vi "Main.vi"(8 "error in (no error)":errorcluster, 9 "Port":u16=4663, 10 "Run External":bool, 11 "Control VI":T1) -> (0 "error out":errorcluster)   [LabVIEW 2024, in "FormulaG.lvlib" / "FormulaG App.lvclass"]
uses:
  FormulaG App.lvclass
  FormulaG-Common/Control VI.ctl
  FormulaG-Common/FormulaG-Common.lvlib
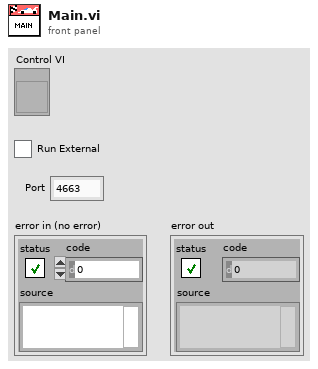
[diagram p1: front panel]
types:
  T1 = typedef "FormulaG-Common.lvlib/Control VI.ctl" = refnum<vi>
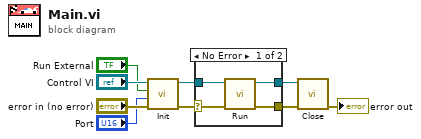
[diagram p0: block diagram]
diagram:
  n1 = call "Init.vi"("error in (no error)"="error in (no error)", "Port"="Port", "Run External"="Run External", "Control VI"="Control VI") -> ("error out"=w9:errorcluster, "FormulaLV App out"=w8:refnum<class "FormulaG App.lvclass">)  [unwired: 6 in]
  n2 = case shown="No Error" w9 {
    selector: w9 -> [w12 w15]
    tunnel: w8 -> [w13 w14]
    tunnel: [w11 w15] -> w7
    tunnel: [w10 w14] -> w6
    frame No Error {
      n3 = call "Run.vi"("error in (no error)"=w12, "FormulaLV App in"=w13) -> ("error out"=w11:errorcluster, "FormulaLV App out"=w10:refnum<class "FormulaG App.lvclass">)  [unwired: 8 in]
    }
    frame Error {
    }
  }
  n4 = call "Close.vi"("error in (no error)"=w7, "FormulaLV App in"=w6) -> ("error out"=→"error out":errorcluster)  [unwired: 9 in]
